vi "Read Mode.vi"(8 "error in":errorcluster, 11 "Electronic Load in":refnum<class "Electronic Load.lvclass">) -> (0 "error out":errorcluster, 2 "Mode":T1, 3 "Electronic Load out":refnum<class "Electronic Load.lvclass">)   [LabVIEW 2019, in "Electronic Load.lvlib" / "Electronic Load.lvclass"]
uses:
  Library/Electronic Load.lvclass
  Custom Controls/E-Load Mode.ctl
  Library/Electronic Load.lvclass/Electronic Load.ctl
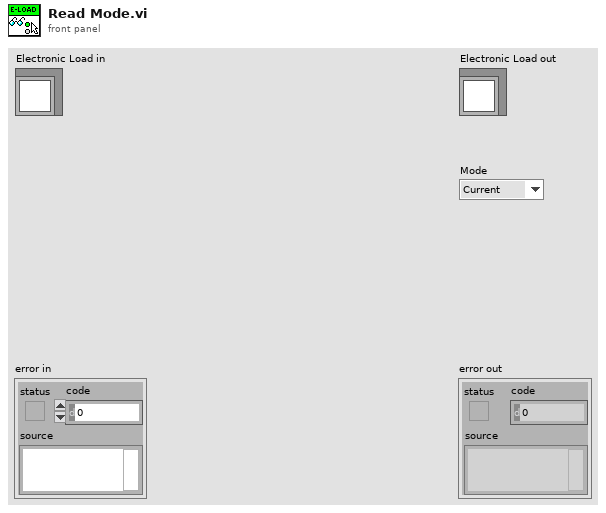
[diagram p1: front panel]
types:
  T1 = typedef "Electronic Load.lvlib/Electronic Load.lvclass/E-Load Mode.ctl" = enum16{"Current", "Resistance", "Voltage"}
  T2 = typedef "Electronic Load.lvlib/Electronic Load.lvclass/E-Load Function.ctl" = cluster{"Mode":T1, "Input Level":dbl, "Output":bool, "Slew Rate":dbl}
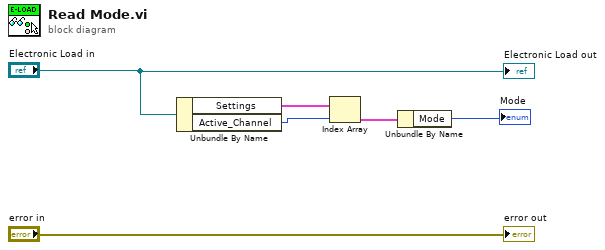
[diagram p0: block diagram]
diagram:
  n1 = Unbundle By Name("Electronic Load in") -> ("Settings"=w4:T2[], "Active_Channel"=w3:u32)
  n2 = Index Array(array=w4, index=w3) -> (element=w2:T2)
  n3 = Unbundle By Name(w2) -> ("Mode"=→"Mode":T1)
  "error out" <- "error in"
  "Electronic Load out" <- "Electronic Load in"
